vi "Show Received Server Messages.vi"(8 "error in (no error)":errorcluster, 10 "String in":refnum<vi>, 11 "Rx String":string) -> (0 "error out":errorcluster, 3 "Received Messages from RT":string)   [LabVIEW 2017]
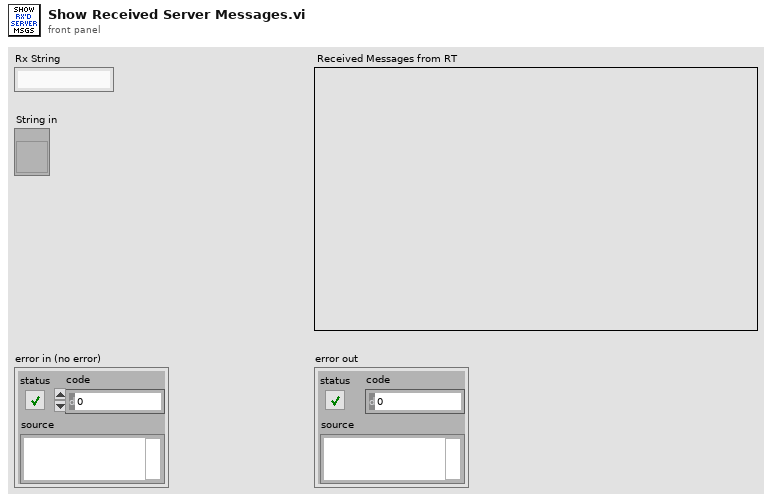
[diagram p1: front panel]
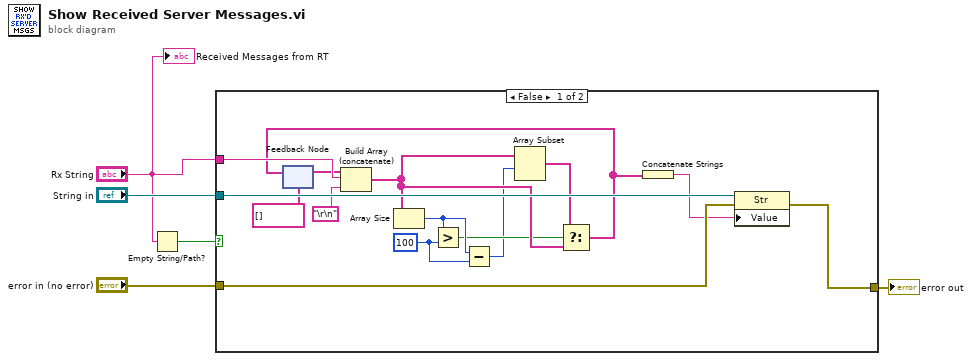
[diagram p0: block diagram]
diagram:
  n1 = Empty String/Path?(string/path="Rx String") -> (empty?=w2:bool)
  n2 = case shown="False" w2 {
    tunnel: "String in" -> [w20 _]
    tunnel: "error in (no error)" -> [w19 w21]
    tunnel: [w18 w21] -> w3
    tunnel: "Rx String" -> [w17 _]
    frame False {
      w8 = 100 ("y")
      n3 = feedback #1(string[] []) -> (w13:string[])
      n4 = Build Array (concatenate)(w13, w17, "\r\n") -> (w12:string[])
      n5 = Array Size(array=w12) -> (size(s)=w15:i32)
      n6 = Greater?(x=w15, y=w8) -> (0:w10:bool)
      n7 = Subtract(x=w15, y=w8) -> (x-y=w9:i32)
      n8 = Array Subset(array=w12, index=w9) -> (w11:string[])  [unwired: 1 in]
      n9 = Select(t=w11, s=w10, f=w12) -> (s? t:f=w16:string[])
      n10 = feedback-in #1(w16) -> ()
      n11 = Concatenate Strings(w16) -> (w6:string)
      n12 = property on="Property Node" class="Str"(reference=w20, error in=w19, "Value"=w6) -> (error out=w18:errorcluster)  [unwired: 1 out]
    }
    frame True {
    }
  }
  "error out" <- w3
  "Received Messages from RT" <- "Rx String"
